vi "VAT_valve_get_status.vi"(8 "error in (no error)":errorcluster, 11 "VAT Valve COM port":refnum<visa-resource-name>) -> (0 "error out":errorcluster, 3 "VAT Valve COM port out":refnum<visa-resource-name>, 4 "Temperature":u32, 5 "Version":dbl, 6 "Status":u32, 7 "Position":u32)   [LabVIEW 2019]
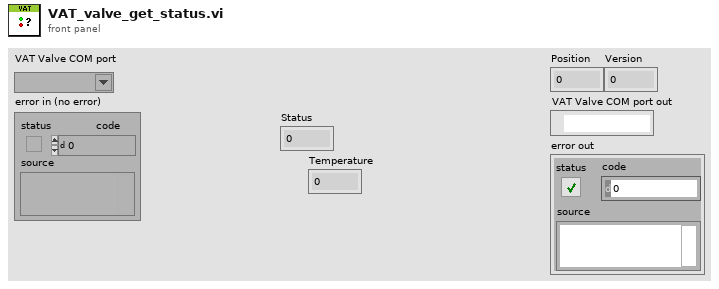
[diagram p1: front panel]
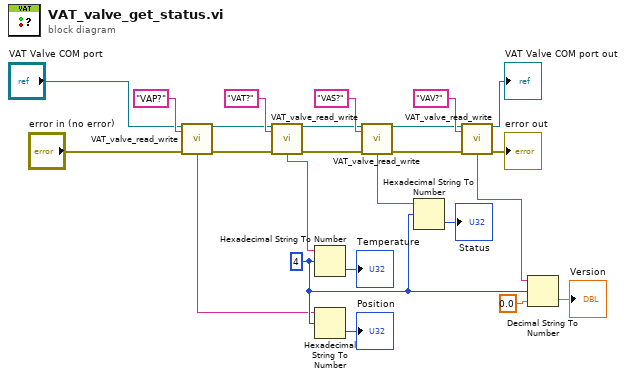
[diagram p0: block diagram]
diagram:
  w21 = 4 ("offset (0)")
  n1 = call "VAT_valve_read_write.vi"("VAT Valve COM port"="VAT Valve COM port", "Write String"="VAP?", "error in (no error)"="error in (no error)") -> ("VAT Valve COM port out"=w12:refnum<visa-resource-name>, "Read String"=w4:string, "error out"=w11:errorcluster)  [unwired: 10 in]
  n2 = call "VAT_valve_read_write.vi"("VAT Valve COM port"=w12, "Write String"="VAT?", "error in (no error)"=w11) -> ("VAT Valve COM port out"=w10:refnum<visa-resource-name>, "Read String"=w3:string, "error out"=w9:errorcluster)  [unwired: 10 in]
  n3 = Hexadecimal String To Number(string=w3, offset=w21) -> (number=→"Temperature":u32)  [unwired: 1 in, 1 out]
  n4 = Hexadecimal String To Number(string=w4, offset=w21) -> (number=→"Position":u32)  [unwired: 1 in, 1 out]
  n5 = call "VAT_valve_read_write.vi"("VAT Valve COM port"=w10, "Write String"="VAS?", "error in (no error)"=w9) -> ("VAT Valve COM port out"=w8:refnum<visa-resource-name>, "Read String"=w2:string, "error out"=w7:errorcluster)  [unwired: 10 in]
  n6 = Hexadecimal String To Number(string=w2, offset=w21) -> (number=→"Status":u32)  [unwired: 1 in, 1 out]
  n7 = call "VAT_valve_read_write.vi"("VAT Valve COM port"=w8, "Write String"="VAV?", "error in (no error)"=w7) -> ("VAT Valve COM port out"=→"VAT Valve COM port out":refnum<visa-resource-name>, "Read String"=w1:string, "error out"=→"error out":errorcluster)  [unwired: 10 in]
  n8 = Decimal String To Number(string=w1, offset=w21, default (0L)=0.0) -> (number=→"Version":dbl)  [unwired: 1 out]
